vi "Test-SharedVariable-ReadQueue.vi"() -> ()   [LabVIEW 2014]
panel:
  out "error IO":errorcluster
  out "读取共享变量":i32(listbox)
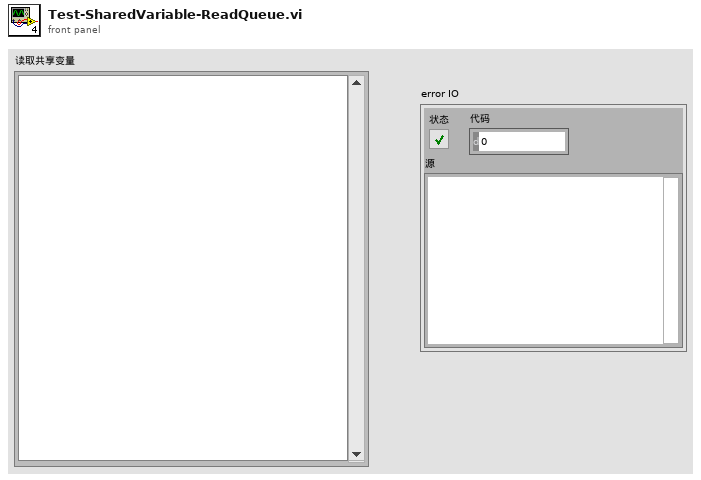
[diagram p1: front panel]
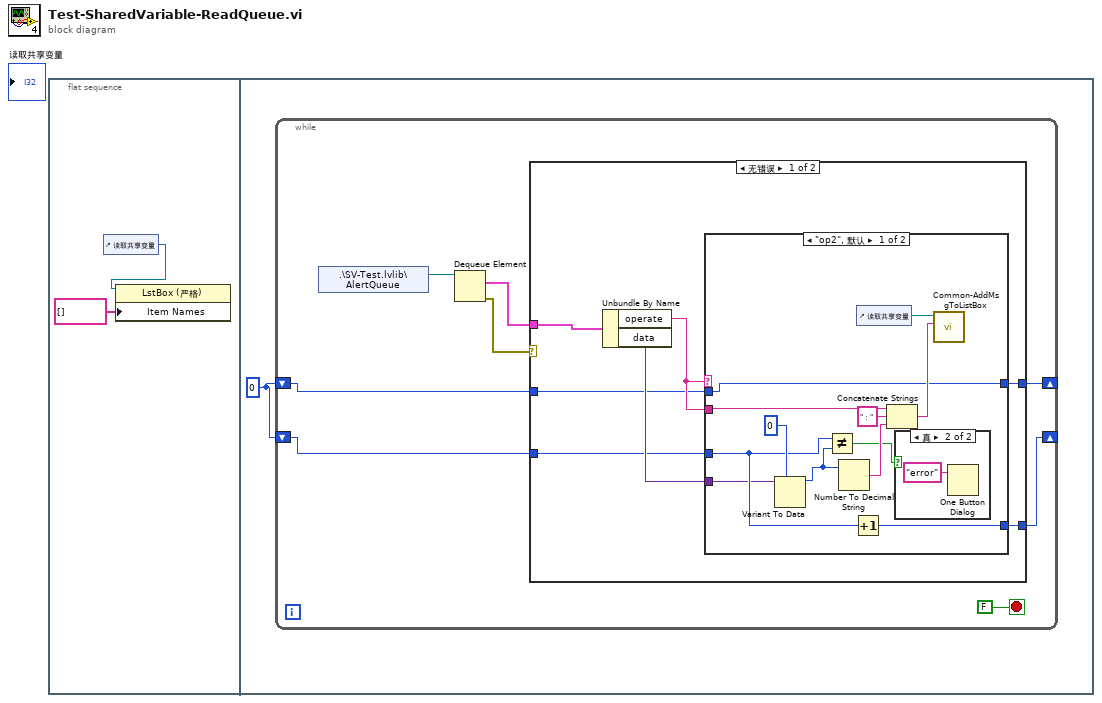
[diagram p0: block diagram]
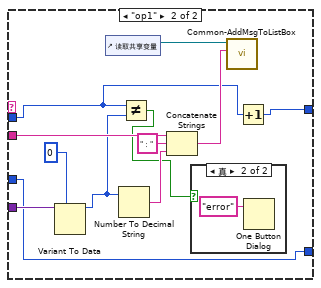
[diagram p3: hidden frame]
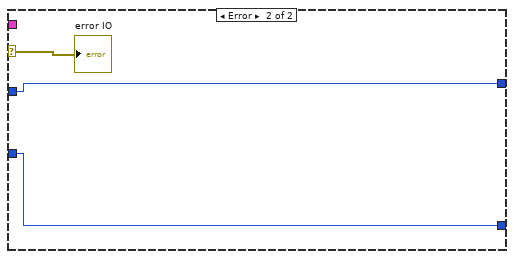
[diagram p5: hidden frame]
diagram:
  n1 = flat-sequence {
    frame #0 {
      n2 = control-ref of="读取共享变量"() -> (w1:refnum<vi>)
      n3 = property class="LstBox (严格)"(reference=w1, "Item Names"=string[] [] ("项名")) -> ()  [unwired: 1 in, 2 out]
    }
    frame #1 {
      w3 = 0
      n4 = while {
        shift-right: [w4] -> _
        shift-left: w3 -> [w7]
        shift-right: [w5] -> _
        shift-left: w3 -> [w6]
        stop <- FALSE stop-if-true
        n5 = shared-variable ".\\SV-Test.lvlib\\AlertQueue"() -> (w10:refnum<queue>)  [unwired: 1 in, 1 out]
        n6 = Dequeue Element(queue=w10) -> (element=w8:cluster{"operate":string, "data":variant}, error out=w9:errorcluster)  [unwired: 2 in, 2 out]
        n7 = case shown="无错误" w9 {
          selector: w9 -> [_ w47]
          tunnel: w8 -> [w18 _]
          tunnel: w7 -> [w15 w46]
          tunnel: w6 -> [w14 w45]
          tunnel: [w13 w45] -> w5
          tunnel: [w12 w46] -> w4
          frame No Error {
            n8 = Unbundle By Name(w18) -> ("operate"=w16:string, "data"=w17:variant)
            n9 = case shown="\"op2\", 默认" w16 {
              tunnel: w16 -> [w25 w42]
              tunnel: w17 -> [w19 w40]
              tunnel: w15 -> [w20 w34]
              tunnel: w14 -> [w22 w32]
              tunnel: [w21 w32] -> w13
              tunnel: [w20 w33] -> w12
              frame "op2", Default {
                n10 = Variant To Data(type=0, Variant=w19) -> (data=w24:i32)  [unwired: 1 in, 1 out]
                n11 = Not Equal?(x=w22, y=w24) -> (x != y?=w23:bool)
                n12 = Number To Decimal String(number=w24) -> (decimal integer string=w27:string)  [unwired: 1 in]
                n13 = Increment(x=w22) -> (x+1=w21:i32)
                n14 = control-ref of="读取共享变量"() -> (w30:refnum<vi>)
                n15 = Concatenate Strings(w25, "：" ("字符串"), w27) -> (w26:string)
                n16 = case shown="真" w23 {
                  frame False {
                  }
                  frame True {
                    n17 = One Button Dialog(message="error" ("消息")) -> ()  [unwired: 1 in, 1 out]
                  }
                }
                n18 = call "Common-AddMsgToListBox.vi"("字符串"=w26, "列表框"=w30) -> ()  [unwired: 10 in]
              }
              frame "op1" {
                n19 = Variant To Data(type=0, Variant=w40) -> (data=w36:i32)  [unwired: 1 in, 1 out]
                n20 = control-ref of="读取共享变量"() -> (w43:refnum<vi>)
                n21 = Number To Decimal String(number=w36) -> (decimal integer string=w38:string)  [unwired: 1 in]
                n22 = Not Equal?(x=w34, y=w36) -> (x != y?=w35:bool)
                n23 = Concatenate Strings(w42, "：" ("字符串"), w38) -> (w37:string)
                n24 = case shown="真" w35 {
                  frame False {
                  }
                  frame True {
                    n25 = One Button Dialog(message="error" ("消息")) -> ()  [unwired: 1 in, 1 out]
                  }
                }
                n26 = call "Common-AddMsgToListBox.vi"("字符串"=w37, "列表框"=w43) -> ()  [unwired: 10 in]
                n27 = Increment(x=w34) -> (x+1=w33:i32)
              }
            }
          }
          frame Error {
            "error IO" <- w47
          }
        }
      }
    }
  }
